vi "Mover4_ikine_with_Kinect.vi"() -> ()   [LabVIEW 2015]
uses:
  <vilib>/MakerHub/KinectOne/Private/Type Defs/Joint Position.ctl
  <vilib>/Utility/miscctls.llb/LV3DPointTypeDef.ctl
  <vilib>/Platform/TimedLoop/XDataNode/timing_clust.ctl
  <vilib>/Platform/TimedLoop/XDataNode/nitl_modes.ctl
  <vilib>/Platform/TimedLoop/XDataNode/wakeup.ctl
  <vilib>/MakerHub/KinectOne/Private/Type Defs/JointType.ctl
  <vilib>/MakerHub/KinectOne/Private/Initialize Image [Color].vi
  <vilib>/MakerHub/KinectOne/Private/kinectRead [BodyFrame].vi
  <vilib>/robotics/Kinematics/Analytical/6R/Type 1/Analytical Inverse Kinematics (6R Type 1).vi
  Microsoft.Kinect
  C:/Program Files (x86)/National Instruments/LabVIEW 2015/vi.lib/MakerHub/KinectOne/Private/Libs/BodyFrameDataInterface.dll
  Program Files (x86)/National Instruments/LabVIEW 2015/vi.lib/MakerHub/KinectOne/Private/Libs/BodyFrameDataInterface.dll
  <vilib>/platform/TimedLoop/XDataNode/XDataNode.xnode
  <vilib>/robotics/Kinematics/Plotting/NI_Robotics_3DKinematics.lvlib
  <vilib>/robotics/Kinematics/NI_Kinematics.lvlib
  <vilib>/MakerHub/KinectOne/KinectOne.lvlib
  <vilib>/robotics/Kinematics/Analytical/NI_Robotics_AnalyticKinematics.lvlib
  <vilib>/robotics/Kinematics/Analytical/6R/Type 1/NI_Robotics_6R Type 1 Serial Arm Class.lvclass
  <vilib>/ptbypt/NI_PtbyPt.lvlib
  <vilib>/Platform/TimedLoop/XDataNode/XDNodeRunTimeDep.lvlib
panel:
  out "Positions":dbl[](array[numeric])
  out "Position not reachable?":bool
  out "Joint Position":T1
  in  "stop":bool
  out "Simulation":refnum<vi>(3d-picture)
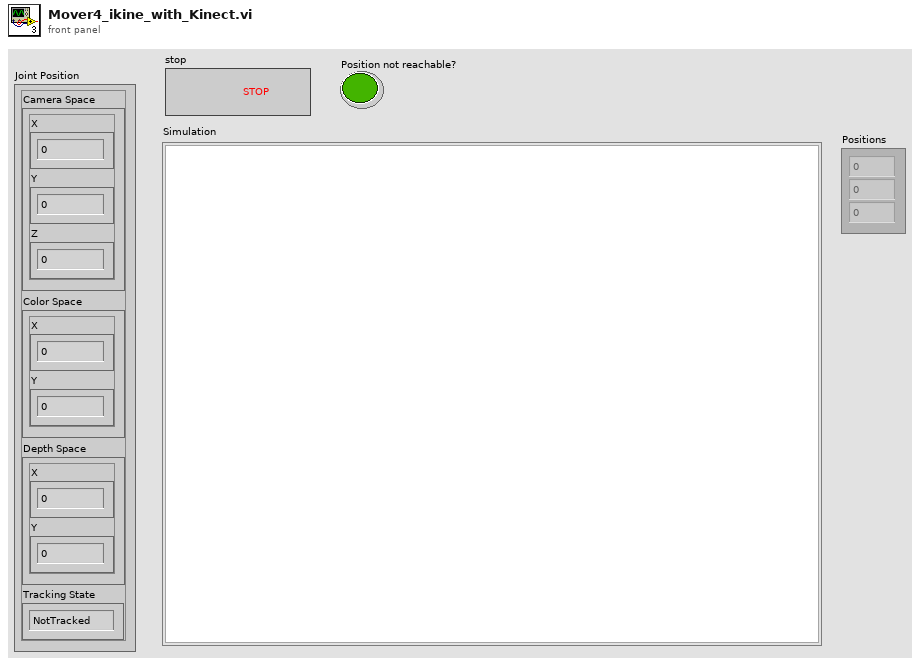
[diagram p1: front panel]
types:
  T1 = typedef "KinectOne.lvlib/Joint Position.ctl" = cluster{"Camera Space":cluster{"X":dbl, "Y":dbl, "Z":dbl}, "Color Space":cluster{"X":dbl, "Y":dbl}, "Depth Space":cluster{"X":dbl, "Y":dbl}, "Tracking State":enum16{"NotTracked", "Inferred", "Tracked"}}
  T2 = typedef "LV3DPointTypeDef.ctl" = cluster{"X":sgl, "Y":sgl, "Z":sgl}
  T3 = typedef "KinectOne.lvlib/KinectSensor References.ctl" = cluster{"KinectSensor":refnum<k24>, "MultiSourceFrameReader":refnum<k24>, "BodyFrameDataInterface":refnum<k24>}
  T4 = typedef "IMAQ Image.ctl" = refnum<image>
  T5 = typedef "XDNodeRunTimeDep.lvlib/timing_clust.ctl" = cluster{"Expected End [f-1]":u64, "Actual End [f-1]":u64, "Finished Late? [f-1]":bool, "Expected End [i-1]":u64, "Actual End [i-1]":u64, "Finished Late? [i-1]":bool, "Expected Start [i]":u64, "Actual Start [i]":u64, "Expected Start [f]":u64, "Actual Start [f]":u64, "Source Name":string, "Structure Name":string, "Period":i64, "Deadline":i64, "Offset":i64, "Start":i64, "Priority":i32, "Timeout":i32, "Mode":T6, "Wakeup Reason":T7, "Error":errorcluster, "Source Type":string, "Secondary Source Type":string, "Global End Time":u64, "Global Start Time":u64, "Frame Duration":u64, "Iteration Duration":u64, "Assigned CPU":i32, "I/O Scan Engine Mode":u32}
  T6 = typedef "XDNodeRunTimeDep.lvlib/nitl_modes.ctl" = enum32{"No Change", "Process missed periods, maintain original phase", "Discard missed periods, maintain original phase", "Process missed periods, ignore original phase", "Discard missed periods, ignore original phase"}
  T7 = typedef "XDNodeRunTimeDep.lvlib/wakeup.ctl" = enum32{"Normal", "Aborted", "Asynchronous wakeup", "Timing source error", "Timed loop error", "Timeout"}
  T8 = typedef "KinectOne.lvlib/JointType.ctl" = enum16{"SpineBase", "SpineMid", "Neck", "Head", "ShoulderLeft", "ElbowLeft", "WristLeft", "HandLeft", "ShoulderRight", "ElbowRight", "WristRight", "HandRight", "HipLeft", "KneeLeft", "AnkleLeft", "FootLeft", "HipRight", "KneeRight", "AnkleRight", "FootRight", "SpineShoulder", "HandTipLeft", "ThumbLeft", "HandTipRight", "ThumbRight"}
  T9 = typedef "KinectOne.lvlib/BodyData.ctl" = cluster{"ClippedEdges":T10, "HandLeftConfidence":T11, "HandLeftState":T12, "HandRightConfidence":T13, "HandRightState":T14, "IsRestricted":bool, "IsTracked":bool, "JointOrientations":refnum<k24>, "Joints":refnum<k24>, "Lean":refnum<k24>, "LeanTrackingState":T15, "TrackingId":u64}
  T10 = typedef "KinectOne.lvlib/ClippedEdges.ctl" = enum16{"None", "Right", "Left", "Top", "Bottom"}
  T11 = typedef "KinectOne.lvlib/HandLeftConfidence.ctl" = enum16{"Low", "High"}
  T12 = typedef "KinectOne.lvlib/HandLeftState.ctl" = enum16{"Unknown", "NotTracked", "Open", "Closed", "Lasso"}
  T13 = typedef "KinectOne.lvlib/HandRightConfidence.ctl" = enum16{"Low", "High"}
  T14 = typedef "KinectOne.lvlib/HandRightState.ctl" = enum16{"Unknown", "NotTracked", "Open", "Closed", "Lasso"}
  T15 = typedef "KinectOne.lvlib/LeanTrackingState.ctl" = enum16{"NotTracked", "Inferred", "Tracked"}
  T16 = typedef "NI_Matrix.lvlib/RealMatrix.ctl" = dbl[][]
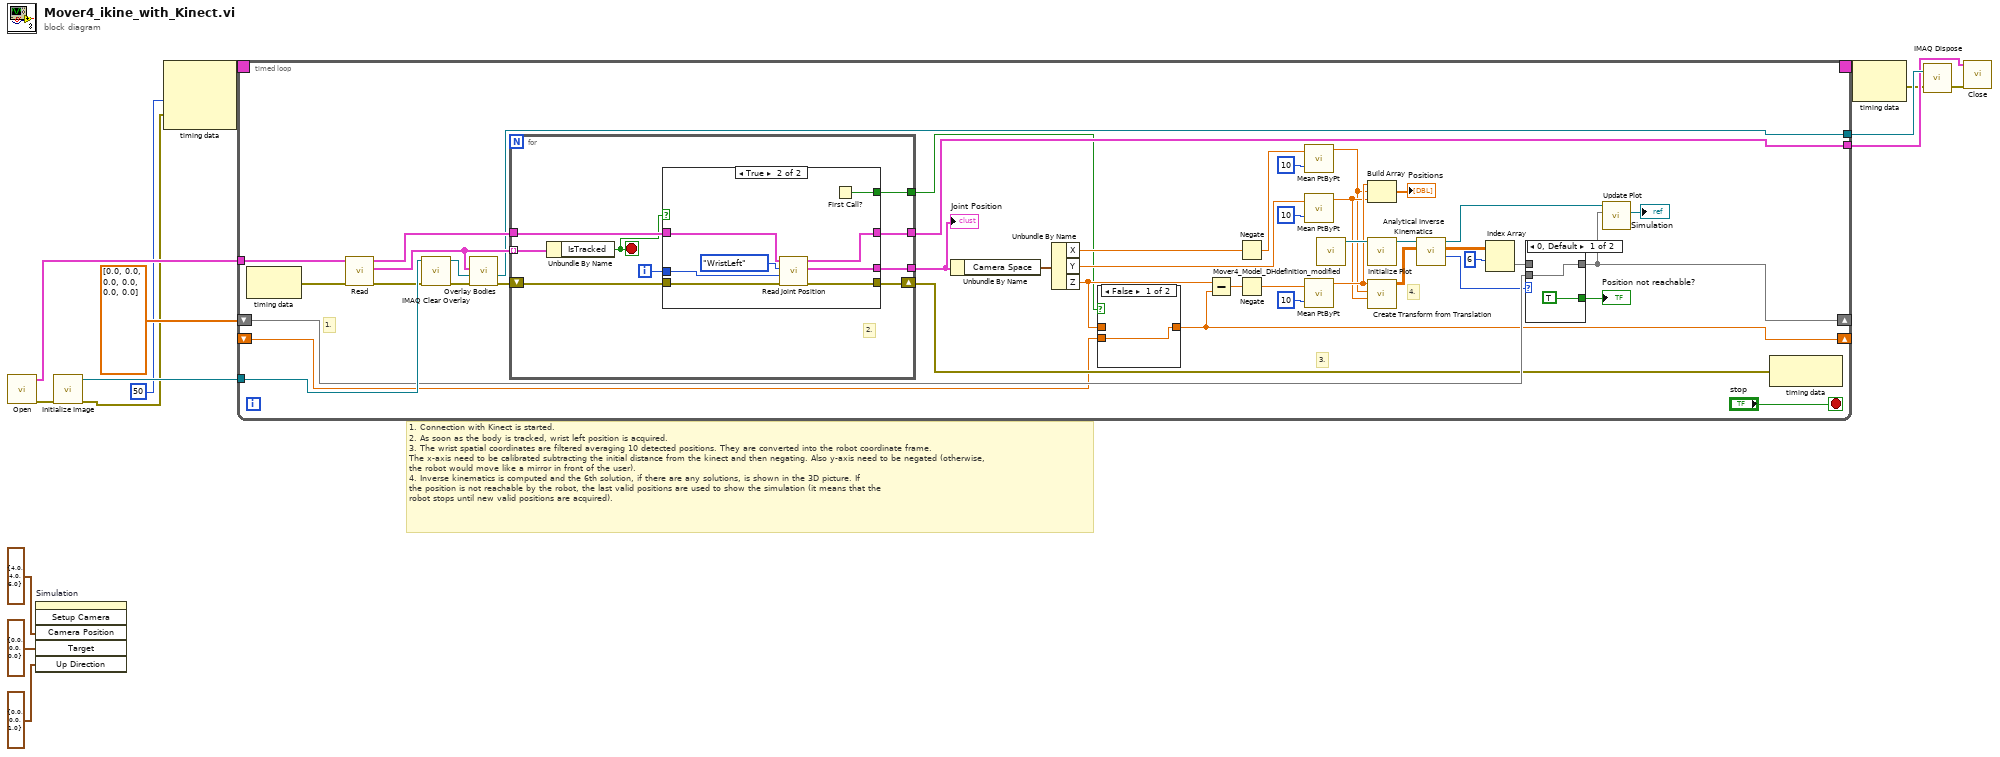
[diagram p0: block diagram]
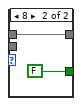
[diagram p3: hidden frame]
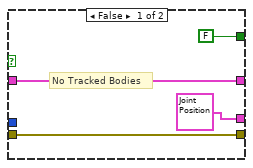
[diagram p4: hidden frame]
diagram:
  # "1. Connection with Kinect is started.\n2. As soon as the body is tracked, wrist left position is acquired.\n3. The wrist spatial coordinates are filtered averaging 10 detected positions. They are converted into the robot coordinate frame.\nThe x-axis need to be calibrated subtracting the initial distance from the kinect and then negating. Also y-axis need to be negated (otherwise,\nthe robot would move like a mirror in front of the user).\n4. Inverse kinematics is computed and the 6th solution, if there are any solutions, is shown in the 3D picture. If\nthe position is not reachable by the robot, the last valid positions are used to show the simulation (it means that the\nrobot stops until new valid positions are acquired)."
  n1 = call <vilib>:"Open.vi"() -> ("Error Out"=w11:errorcluster, "KinectSensor References out"=w10:T3)  [unwired: 10 in]
  n2 = invoke on="Simulation" class="SceneGraphDisp (strict)" method="Setup Camera"("Camera Position"=T2 {"X"=4.0, "Y"=4.0, "Z"=6.0}, "Target"=T2 {"X"=0.0, "Y"=0.0, "Z"=0.0}, "Up Direction"=T2 {"X"=0.0, "Y"=0.0, "Z"=1.0}) -> ()  [unwired: 3 in, 6 out]
  n3 = call-poly <vilib>:"Initialize Image.vi"("Error In"=w11) -> ("Error Out"=w2:errorcluster, "Color Image"=w9:T4)  [unwired: 9 in]
  n4 = node-c288(i64 50 ("Period"), w2) -> (w5:T5)  [unwired: 1 in]
  n5 = timed-loop {
    shift-right: [w36] -> _
    shift-left: dbl[] [0.0, 0.0, 0.0, 0.0, 0.0, 0.0] ("current joint positions") -> [w41]
    tunnel: w10 -> [w55]
    tunnel: w9 -> [w54]
    tunnel: [w48] -> w8
    tunnel: [w46] -> w6
    timing: w5 -> [_]
    timing-out: [_] -> w4
    shift-right: [w18] -> _
    shift-left: _ -> [w17]
    stop <- "stop" stop-if-true
    # "4."
    # "3."
    # "1."
    n6 = node-c288() -> (w21:errorcluster)  [unwired: 1 in]
    n7 = call-poly <vilib>:"Read.vi"("error in (no error)"=w21, "KinectSensor References in"=w55) -> ("error out"=w53:errorcluster, "Body Data"=w50:T9[], "KinectSensor References out"=w49:T3)  [unwired: 7 in]
    n8 = call "IMAQ Clear Overlay"("error in (no error)"=w53, "Image"=w54) -> ("error out"=w51:errorcluster, "Image Out"=w52:T4)  [unwired: 8 in]
    n9 = call <vilib>:"Overlay Bodies.vi"("Error In"=w51, "Image"=w52, "Body Data"=w50) -> ("Error Out"=w47:errorcluster, "Image Out"=w48:T4)  [unwired: 7 in]
    n10 = for {
      tunnel: [w76] -> w46
      tunnel: w49 -> [w75]
      tunnel: [w74] -> w45
      shift-right: [w77] -> w20
      shift-left: w47 -> [w78]
      tunnel: w50 -> [w73] mode=indexing
      tunnel: [w70] -> w16
      i -> [w71]
      stop <- w72 stop-if-true
      # "2."
      n11 = Unbundle By Name(w73) -> ("IsTracked"=w72:bool)
      n12 = case shown="True" w72 {
        tunnel: w78 -> [w81 w90]
        tunnel: [w81 w89] -> w77
        tunnel: [w82 w88] -> w76
        tunnel: w75 -> [w82 w87]
        tunnel: [T1 {"Camera Space"={"X"=0.0, "Y"=0.0, "Z"=0.0}, "Color Space"={"X"=0.0, "Y"=0.0}, "Depth Space"={"X"=0.0, "Y"=0.0}, "Tracking State"=enum."NotTracked"} ("Joint Position") w85] -> w74
        tunnel: w71 -> [_ w84]
        tunnel: [FALSE w83] -> w70
        frame False {
          # "No Tracked Bodies"
        }
        frame True {
          n13 = call <vilib>:"Read Joint Position.vi"("Error In"=w90, "Body Index"=w84, "JointType"=JointType."WristLeft", "KinectSensor References"=w87) -> ("Error Out"=w89:errorcluster, "Joint Position"=w85:T1, "KinectSensor References"=w88:T3)  [unwired: 4 in, 1 out]
          n14 = First Call?() -> (First Call?: T/F=w83:bool)
        }
      }
    }
    "Joint Position" <- w45
    n15 = Unbundle By Name(w45) -> ("Camera Space"=w44:cluster{"X":dbl, "Y":dbl, "Z":dbl})
    n16 = Unbundle By Name(w44) -> ("X"=w33:dbl, "Y"=w27:dbl, "Z"=w19:dbl)
    n17 = case shown="False" w16 {
      tunnel: w19 -> [_ w60]
      tunnel: [w59 w60] -> w18
      tunnel: w17 -> [w59 _]
      frame False {
      }
      frame True {
      }
    }
    n18 = Subtract(x=w19, y=w18) -> (x-y=w31:dbl)
    n19 = Negate(x=w33) -> (-x=w24:dbl)
    n20 = Negate(x=w31) -> (-x=w30:dbl)
    n21 = call <vilib>:"Mean PtByPt.vi"("x"=w24, "sample length"=10) -> ("mean"=w23:dbl)  [unwired: 2 in, 1 out]
    n22 = call <vilib>:"Mean PtByPt.vi"("x"=w27, "sample length"=10) -> ("mean"=w26:dbl)  [unwired: 2 in, 1 out]
    n23 = call <vilib>:"Mean PtByPt.vi"("x"=w30, "sample length"=10) -> ("mean"=w29:dbl)  [unwired: 2 in, 1 out]
    n24 = call "Mover4_Model_DHdefinition_modified.vi"() -> ("serial arm out"=w43:refnum<class "NI_Robotics_6R Type 1 Serial Arm Class.lvclass">)  [unwired: 10 in, 1 out]
    n25 = Build Array(w29, w23, w26) -> (→"Positions":dbl[])
    n26 = call <vilib>:"Initialize Plot.vi"("serial arm in"=w43) -> ("serial arm out"=w42:refnum<class "NI_Robotics_6R Type 1 Serial Arm Class.lvclass">)  [unwired: 9 in, 1 out]
    n27 = call <vilib>:"Create Transform from Translation.vi"("z"=w26, "y"=w23, "x"=w29) -> ("transform"=w40:T16)  [unwired: 8 in]
    n28 = call-poly <vilib>:"Analytical Inverse Kinematics.vi"("end effector transform"=w40, "6R type 1 serial arm in"=w42) -> ("number of valid solutions"=w35:i32, "joint positions"=w39:T16, "6R type 1 serial arm out"=w57:refnum<class "NI_Robotics_6R Type 1 Serial Arm Class.lvclass">)  [unwired: 6 in, 1 out]
    n29 = Index Array(array=w39, index (row)=6) -> (element=w37:dbl[])  [unwired: 1 in]
    n30 = case shown="0, Default" w35 {
      tunnel: w41 -> [w67 _]
      tunnel: w37 -> [_ w69]
      tunnel: [w67 w69] -> w36
      tunnel: [TRUE FALSE] -> w34
      frame 0, Default {
      }
      frame 8 {
      }
    }
    "Position not reachable?" <- w34
    n31 = call <vilib>:"Update Plot.vi"("joint positions"=w36, "serial arm in"=w57) -> ("serial arm scene"=→"Simulation":refnum<vi>)  [unwired: 7 in, 2 out]
    n32 = node-c288(w20) -> ()  [unwired: 1 out]
  }
  n33 = node-c288(w4) -> (w1:errorcluster)
  n34 = call "IMAQ Dispose"("Image"=w8, "error in (no error)"=w1) -> ("error out"=w7:errorcluster)  [unwired: 4 in]
  n35 = call <vilib>:"Close.vi"("Error In"=w7, "KinectSensor References"=w6) -> ()  [unwired: 9 in, 1 out]
